vi "ziExample-Module-SweepUtility.vi"() -> ()   [LabVIEW 2016]
doc: "Control a Zurich instrument device via the LabOne Labview API. \nRequirements: Zurich Instruments MFLI, HF2 or UHFLI \nThis example shows how to start a sweeper module and retrieve data in an interactive vi.\n\n© Zurich Instruments AG, www.zhinst.com"
uses:
  <instrlib>/Zurich Instruments LabOne/Public/Modules/ziTypeModEnum.ctl
  <instrlib>/Zurich Instruments LabOne/Public/Modules/ziModSetValueBinary.vi
  <instrlib>/Zurich Instruments LabOne/Public/Modules/ziModGetDoubleData.vi
  <instrlib>/Zurich Instruments LabOne/Public/Modules/ziModGetByteArray.vi
  <instrlib>/Zurich Instruments LabOne/Public/Modules/ziModGetSweeperData.vi
  <instrlib>/Zurich Instruments LabOne/Public/Modules/ziModSetValueDouble.vi
  <instrlib>/Zurich Instruments LabOne/Zurich Instruments LabOne.lvlib
panel:
  out "Error Out":errorcluster
  in  "Host:port (optional)":string
  out "Mod subs paths":string[](array[string])
  in  "demods/x/sample":bool[](array[boolean])=[TRUE]
  in  "sweep/xmapping":i32(ring)=1 caption="X Mapping" items=["Linear", "Log"]
  in  "sweep/loopcount":i32=2 caption="Loop Count (#)" min=1 max=66000
  in  "sweep/order":u16(ring) caption="Order" items=["Current Setting", "6 dB/oct", "12 dB/oct", "18 dB/oct", "24 dB/oct", "30 dB/oct", "36 dB/oct", "42 dB/oct", "48 dB/oct"]
  out "Progress":dbl(slide) scale=0.0..1.0
  out "Finished?":bool
  in  "sweep/settling/inaccuracy":dbl caption="Inaccuracy" format="%#_5p"
  in  "sweep/scan":u16(ring) caption="Scan" items=["Sequential", "Binary", "Bidirectional"]
  in  "sweep/settling/time":dbl caption="Settling (s)" format="%#_5p"
  in  "sweep/bandwidth":dbl caption="BW (Hz)" format="%#_5p"
  in  "sweep/bandwidthcontrol":u16(ring) caption="BW Control" items=["Manual", "Fixed", "Automatic"]
  in  "sweep/phaseunwrap":bool caption="Phase Unwrap"
  in  "sweep/maxbandwidth":dbl caption="Max BW (Hz)" format="%#_5p"
  in  "sweep/averaging/tc":dbl caption="Averaging TCs" format="%#_5p"
  in  "sweep/averaging/sample":dbl caption="Averaging Samples" format="%#_5p"
  in  "Stop Sweep":bool
  in  "sweep/endless":bool caption="Endless"
  in  "start_act":bool
  in  "sweep/gridnode":string="oscs/0/freq"
  in  "sweep/omegasuppression":dbl caption="Omega Suppression (dB)" format="%#_5p"
  in  "sweep/sincfilter":bool caption="Sinc"
  in  "sweep/samplecount":i32=2 caption="Points (#)" min=2 max=66000
  in  "sweep/stop":dbl caption="Stop (Hz)" format="%_5p"
  in  "sweep/start":dbl caption="Start (Hz)" format="%_5p"
  in  "stop":bool
  in  "Address":string="DEV" caption="Device ID"
  out "Selected Device":string
  out "Sweeper Phase":cluster{"grid":dbl[], "phase":dbl[]}[](graph)
  out "Sweeper R":cluster{"grid":dbl[], "phase":dbl[]}[](graph)
  # "ziExample-SweepModul.vi\nRequirements: HF2LI, UHFLI or MFLI\nsee block diagram for VI description"
  # "Tested Devices:\n- MFLI\n- HF2LI\n- UHFLI"
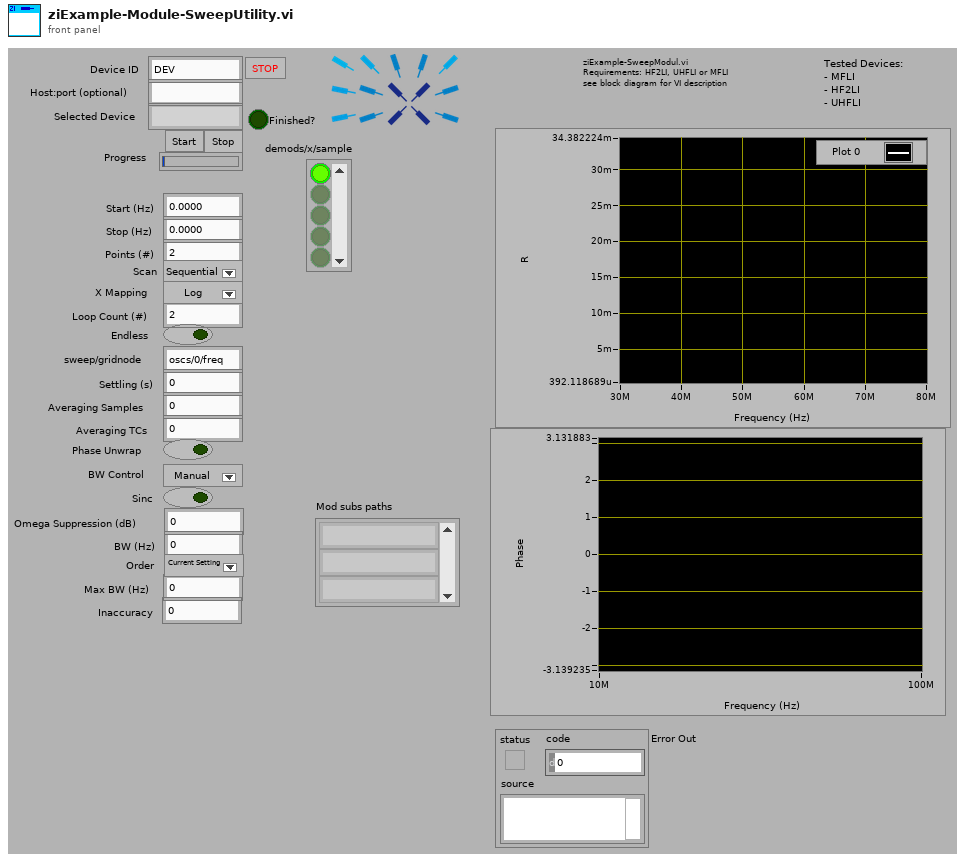
[diagram p1: front panel]
types:
  T1 = typedef "Zurich Instruments LabOne.lvlib/ziTypeModEnum.ctl" = u16
  T2 = typedef "Zurich Instruments LabOne.lvlib/ziTypeHandle.ctl" = cluster{"handleValid":bool, "Conn":u64, "Path Prefix":string, "Handle":u64, "Connected":bool, "Clockbase(s)":dbl}
  T3 = typedef "Zurich Instruments LabOne.lvlib/ziTypeModHandle.ctl" = cluster{"handleValid":bool, "Conn":u64, "ModHandle":u64, "moduleID":string, "Path Prefix":string}
  T4 = cluster{"Label.Text":string, "Label.Text 2":string}
  T5 = typedef "Zurich Instruments LabOne.lvlib/ziTypeModResults.ctl" = cluster{"PathArray":string[], "ValueType":T6, "NoOfResults":u64, "ziGenericHeader":T7[]}
  T6 = typedef "Zurich Instruments LabOne.lvlib/ziTypePollType.ctl" = enum16{"NONE", "DOUBLE_DATA", "INTEGER_DATA", "DEMOD_SAMPLE", "SCOPE_WAVE_HF2", "AUXIN_SAMPLE", "DIO_SAMPLE", "BYTE_ARRAY", "PWA_WAVE", "9", "10", "11", "12", "13", "14", "15", "TREE_CHANGE_DEPRI", "17", "ERROR", "19", "20", "21", "22", "23", "24", "25", "26", "27", "28", "29", "30", "31", "DOUBLE_DATA_TS", "INTEGER_DATA_TS", "34", "SCOPE_WAVE", "SCOPE_WAVE_EX", "37", "BYTE_ARRAY_TS", "39", "40", "41", "42", "43", "44", "45", "CNT_DATA", "47", "TREE_CHANGE", "49", "50", "51", "52", "53", "54", "55", "56", "57", "58", "59", "60", "61", "62", "63", "SWEEPER_DATA", "SPECTRUM_DATA", "ADVISOR_DATA", "VECTOR_DATA", "IMP_DATA"}
  T7 = typedef "Zurich Instruments LabOne.lvlib/ziTypeModGenericHeader.ctl" = cluster{"HeaderType":enum8{"HEADER_TYPE_NONE", "HEADER_TYPE_SWTRIGGER", "HEADER_TYPE_SWEEPER"}, "SampleFormat":u8, "SystemTime":timestamp, "CreatedTimeStamp":u64, "ChangedTimeStamp":u64, "Flags":u32, "ChunkSizeBytes":u64, "Name":string, "Status":u32, "GroupIndex":u32, "Color":u32, "ActiveRow":u32, "TriggerNumber":u64, "GridRows":u32, "GridCols":u32, "GridMode":u32, "GridOperation":u32, "GridDirection":u32, "GridRepetitions":u32, "GridColDelta":dbl, "GridColOffset":dbl, "GridRowDelta":dbl, "GridRowOffset":dbl, "Bandwidth":dbl, "Center":dbl, "Nenbw":dbl}
  T8 = typedef "Zurich Instruments LabOne.lvlib/ziTypeByteArray.ctl" = cluster{"Timestamp (ticks)":u64[], "string":string[]}
  T9 = typedef "Zurich Instruments LabOne.lvlib/ziTypeModSweeperDemodWave.ctl" = cluster{"timestamp":u64, "sampleCount":u64, "flags":u8, "sampleFormat":u8, "sweepMode":u8, "bandwidthMode":u8, "count":u64[], "settimestamp":u64[], "nexttimestamp":u64[], "grid":dbl[], "bandwidth":dbl[], "tc":dbl[], "tcmeas":dbl[], "settling":dbl[], "x":dbl[], "xstddev":dbl[], "xpwr":dbl[], "y":dbl[], "ystddev":dbl[], "ypwr":dbl[], "r":dbl[], "rstddev":dbl[], "rpwr":dbl[], "phase":dbl[], "phasestddev":dbl[], "phasepwr":dbl[], "frequency":dbl[], "frequencystddev":dbl[], "frequencypwr":dbl[], "auxin0":dbl[], "auxin0stddev":dbl[], "auxin0pwr":dbl[], "auxin1":dbl[], "auxin1stddev":dbl[], "auxin1pwr":dbl[]}
  T10 = cluster{"Label.Text":string, "Label.Text 2":string}[]
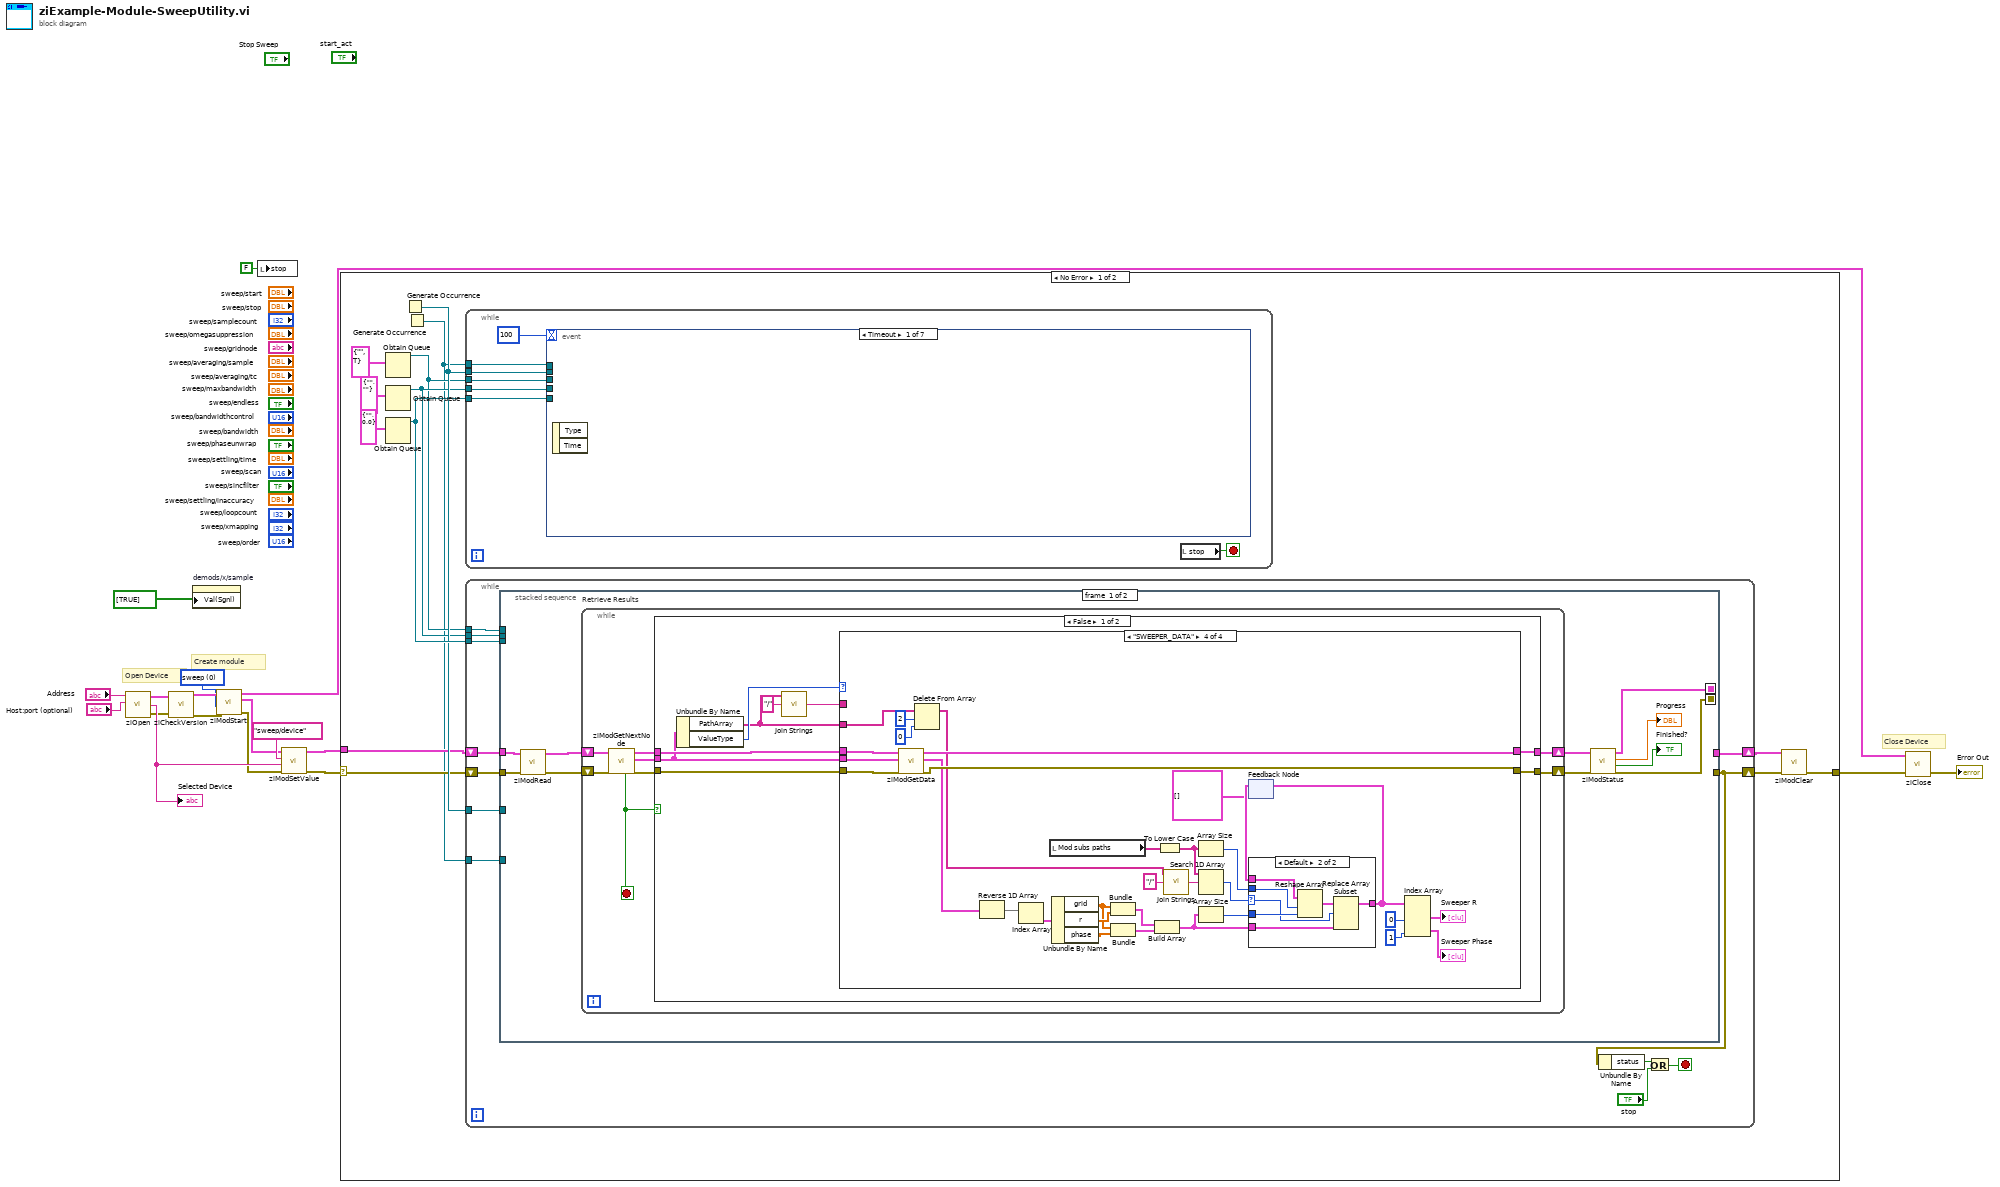
[diagram p0: block diagram]
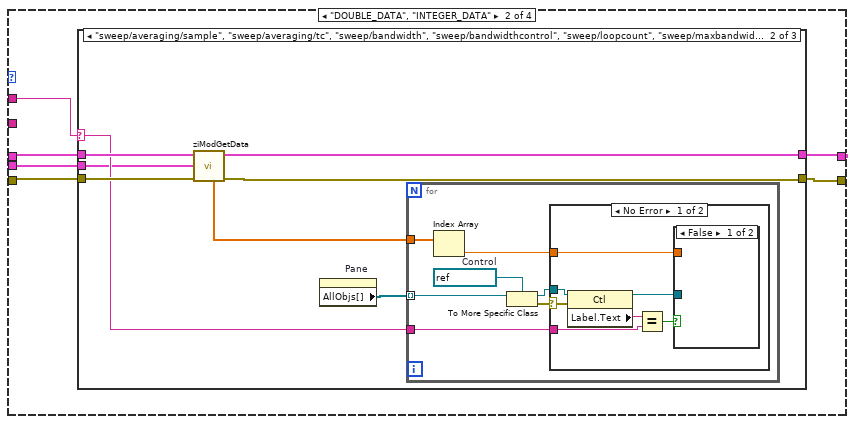
[diagram p3: hidden frame]
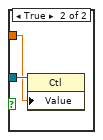
[diagram p5: hidden frame]
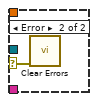
[diagram p6: hidden frame]
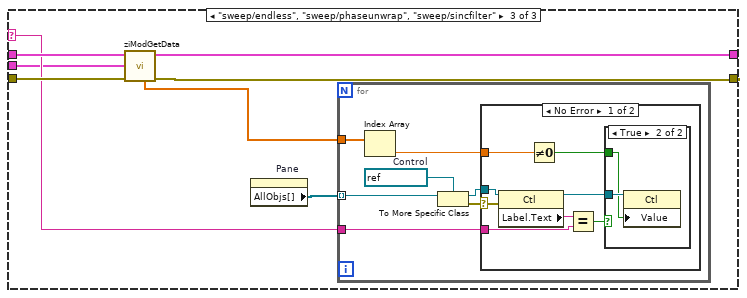
[diagram p7: hidden frame]
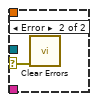
[diagram p9: hidden frame]
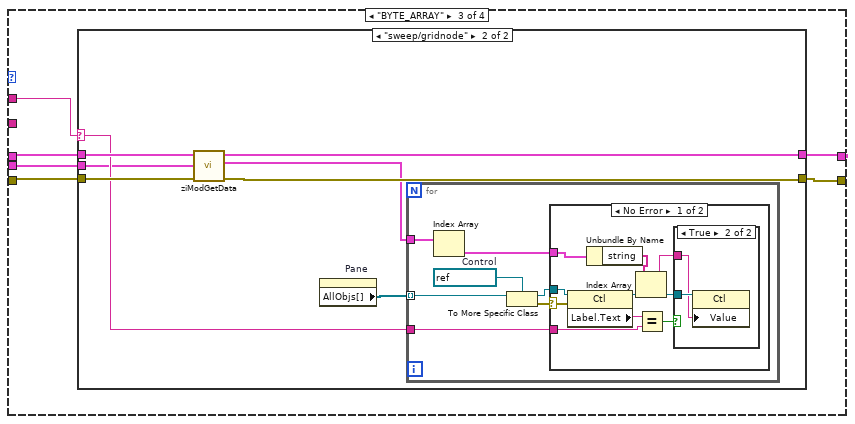
[diagram p10: hidden frame]
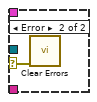
[diagram p13: hidden frame]
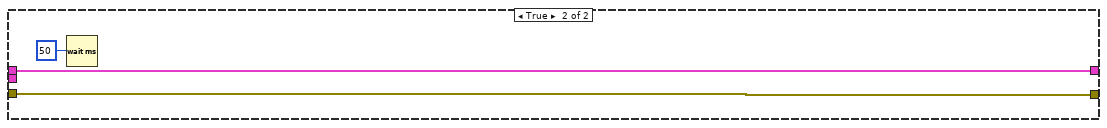
[diagram p15: hidden frame]
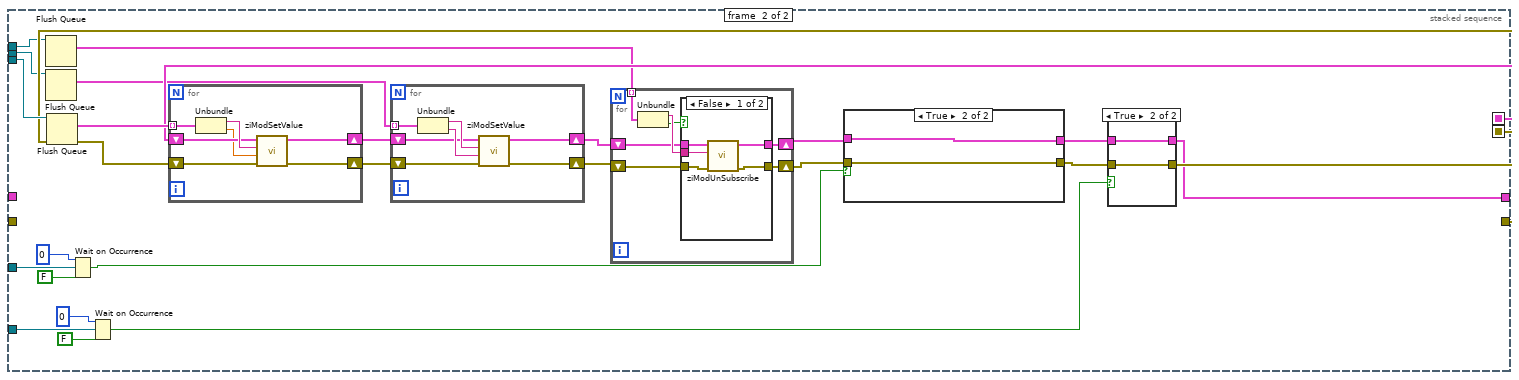
[diagram p16: hidden frame]
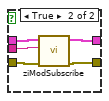
[diagram p17: hidden frame]
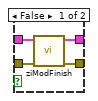
[diagram p18: hidden frame]
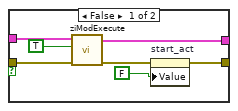
[diagram p19: hidden frame]
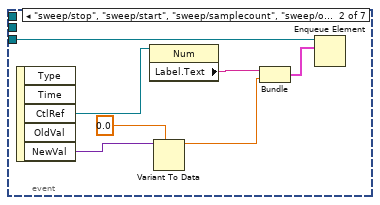
[diagram p20: hidden frame]
diagram:
  w1 = T1 0 items=["sweep", "scopeModule", "dataAcquisitionModule", "pidAdvisor", "awgModule", "impedanceModule", "multiDeviceSyncModule", "zoomFFT", "trigger", "deviceSettings", "record"] ("module Id")
  # "Close Device"
  # "Create module"
  # "Open Device"
  n1 = call <instrlib>:"ziOpen.vi"("Hostname obsolete (auto)"="Host:port (optional)", "Address"="Address") -> ("Error Out"=w5:errorcluster, "Selected Device"=w17:string, "HandleOut"=w6:T2)  [unwired: 1 in, 1 out]
  "Selected Device" <- w17
  n2 = call <instrlib>:"ziCheckVersion.vi"("Handle In"=w6, "Error In"=w5) -> ("Handle Out"=w4:T2, "Error Out"=w3:errorcluster)  [unwired: 11 in, 1 out]
  n3 = property on="demods/x/sample" class="Arr (strict)"("Val(Sgnl)"=bool[] [TRUE] ("Value (Signaling)")) -> ()  [unwired: 2 in, 2 out]
  n4 = call <instrlib>:"ziModStart.vi"("Error In"=w3, "module Id"=w1, "Handle In"=w4) -> ("Error Out"=w15:errorcluster, "ModHandle Out"=w13:T3, "Handle Out"=w16:T2)  [unwired: 6 in]
  n5 = local write "stop"(FALSE ("Stop")) -> ()
  n6 = call-poly <instrlib>:"ziModSetValue.vi"("Error In"=w15, "Data"=w17, "Path"="sweep/device", "ModHandle In"=w13) -> ("Error Out"=w10:errorcluster, "ModHandle Out"=w12:T3)  [unwired: 6 in]
  n7 = case shown="No Error" w10 {
    selector: w10 -> [w24 w329]
    tunnel: [w31 w329] -> w18
    tunnel: w12 -> [w25 _]
    frame No Error {
      n8 = Obtain Queue(element data type=cluster{"Label.Text":string, bool} {"Label.Text"="", TRUE} ("output cluster")) -> (queue out=w20:refnum<queue>)  [unwired: 4 in, 2 out]
      n9 = Obtain Queue(element data type=T4 {"Label.Text"="", "Label.Text 2"=""} ("output cluster")) -> (queue out=w21:refnum<queue>)  [unwired: 4 in, 2 out]
      n10 = Obtain Queue(element data type=cluster{"Label.Text":string, "sweep/stop":dbl} {"Label.Text"="", "sweep/stop"=0.0} ("output cluster")) -> (queue out=w27:refnum<queue>)  [unwired: 4 in, 2 out]
      n11 = Generate Occurrence() -> (w26:refnum<k4>)
      n12 = Generate Occurrence() -> (w19:refnum<k4>)
      n13 = while {
        tunnel: w27 -> [w287]
        tunnel: w26 -> [w286]
        tunnel: w21 -> [w285]
        tunnel: w20 -> [w284]
        tunnel: w19 -> [w283]
        stop <- w289 stop-if-true
        n14 = event shown="[0] Timeout" {
          selector: _ -> [_ _ _ _ _ _ _]
          dyn-events: _ -> [_ _ _ _ _ _ _]
          timeout: 100 -> [_ _ _ _ _ _ _]
          tunnel: w287 -> [_ w293 w297 _ _ _ _]
          tunnel: w286 -> [_ _ _ _ w310 _ _]
          tunnel: w285 -> [_ _ _ w307 _ _ _]
          tunnel: w284 -> [_ _ _ _ _ w311 _]
          tunnel: w283 -> [_ _ _ _ _ _ w328]
          event Timeout {
            n15 = event-data() -> ()  [unwired: 1 in, 2 out]
          }
          event "sweep/stop", "sweep/start", "sweep/samplecount", "sweep/omegasuppression", "sweep/averaging/sample", "sweep/averaging/tc", "sweep/maxbandwidth", "sweep/bandwidthcontrol", "sweep/settling/time", "sweep/scan", "sweep/loopcount", "sweep/xmapping", "sweep/order": Value Change {
            n16 = event-data() -> ("CtlRef"=w294:refnum<vi>, "NewVal"=w295:variant)  [unwired: 1 in, 3 out]
            n17 = property class="Num"(reference=w294) -> ("Label.Text"=w292:string)  [unwired: 1 in, 2 out]
            n18 = Variant To Data(type=0.0 ("sweep/stop"), Variant=w295) -> (data=w291:dbl)  [unwired: 1 in, 1 out]
            n19 = Bundle("Label.Text"=w292, "sweep/stop"=w291) -> (w290:cluster{"Label.Text":string, "sweep/stop":dbl})  [unwired: 1 in]
            n20 = Enqueue Element(queue=w293, element=w290) -> ()  [unwired: 2 in, 3 out]
          }
          event "sweep/phaseunwrap", "sweep/endless", "sweep/sincfilter": Value Change {
            n21 = event-data() -> ("CtlRef"=w302:refnum<vi>, "NewVal"=w299:bool)  [unwired: 1 in, 3 out]
            n22 = property class="Bool (strict)"(reference=w302) -> ("Label.Text"=w301:string)  [unwired: 1 in, 2 out]
            n23 = Boolean To (0,1)(Boolean=w299) -> (0, 1=w300:i16)
            n24 = Bundle("Label.Text"=w301, w300) -> (w298:cluster{"Label.Text":string, i16})  [unwired: 1 in]
            n25 = Enqueue Element(queue=w297, element=w298) -> ()  [unwired: 2 in, 3 out]
          }
          event "sweep/gridnode": Value Change {
            n26 = event-data() -> ("CtlRef"=w309:refnum<vi>, "NewVal"=w303:string)  [unwired: 1 in, 3 out]
            n27 = property class="Str"(reference=w309) -> ("Label.Text"=w304:string)  [unwired: 1 in, 2 out]
            n28 = Variant To Data(type="", Variant=w303) -> (data=w308:string)  [unwired: 1 in, 1 out]
            n29 = Bundle("Label.Text"=w304, w308) -> (w305:cluster{"Label.Text":string, string})  [unwired: 1 in]
            n30 = Enqueue Element(queue=w307, element=w305) -> ()  [unwired: 2 in, 3 out]
          }
          event "start_act": Value Change {
            n31 = event-data() -> ()  [unwired: 1 in, 5 out]
            n32 = Set Occurrence(w310) -> ()
          }
          event "demods/x/sample": Value Change {
            n33 = event-data() -> ()  [unwired: 1 in, 5 out]
            n34 = for {
              tunnel: "demods/x/sample" -> [w320] mode=indexing
              tunnel: "demods/%d/sample" -> [w319]
              shift-right: [w321] -> w312
              shift-left: string[] [] ("Mod subs paths") -> [w322]
              tunnel: w311 -> [w317]
              i -> [w323]
              n35 = Format Into String(format string=w319, w323) -> (resulting string=w316:string)  [unwired: 2 in, 1 out]
              n36 = Bundle(w316, "Boolean"=w320) -> (w318:cluster{string, "Boolean":bool})  [unwired: 1 in]
              n37 = case shown="False" w320 {
                tunnel: w322 -> [w324 w327]
                tunnel: w316 -> [_ w326]
                tunnel: [w324 w325] -> w321
                frame False {
                }
                frame True {
                  n38 = Build Array (concatenate)(w327, w326) -> (w325:string[])
                }
              }
              n39 = Enqueue Element(queue=w317, element=w318) -> ()  [unwired: 2 in, 3 out]
            }
            "Mod subs paths" <- w312
          }
          event "Stop Sweep": Value Change {
            n40 = event-data() -> ()  [unwired: 1 in, 5 out]
            n41 = Set Occurrence(w328) -> ()
          }
        }
        n42 = local read "stop"() -> (w289:bool)
      }
      n43 = while {
        shift-right: [w36] -> w30
        shift-left: w25 -> [w40]
        shift-right: [w35] -> w29
        shift-left: w24 -> [w43]
        tunnel: w27 -> [w42]
        tunnel: w26 -> [w41]
        tunnel: w21 -> [w39]
        tunnel: w20 -> [w38]
        tunnel: w19 -> [w37]
        stop <- w32 stop-if-true
        n44 = stacked-sequence {
          seq-local: [w46 _] -> [_ w230]
          seq-local: [w44 _] -> [_ w229]
          tunnel: w43 -> [w53 _]
          tunnel: w42 -> [_ w236]
          tunnel: w41 -> [_ w234]
          tunnel: w40 -> [w45 _]
          tunnel: w39 -> [_ w227]
          tunnel: w38 -> [_ w226]
          tunnel: w37 -> [_ w216]
          tunnel: [_ w212] -> w35
          tunnel: [_ w211] -> w36
          frame #0 {
            n45 = call <instrlib>:"ziModRead.vi"("error in"=w53, "ziModHandle In"=w45) -> ("error out"=w52:errorcluster, "ziModHandle Out"=w51:T3)  [unwired: 8 in]
            n46 = while "Retrieve Results" {
              shift-right: [w58] -> w50
              shift-left: w51 -> [w60]
              shift-right: [w57] -> w48
              shift-left: w52 -> [w61]
              stop <- w54 stop-if-true
              n47 = call <instrlib>:"ziModGetNextNode.vi"("Error In"=w61, "ModHandle In"=w60) -> ("Error Out"=w55:errorcluster, "ModResults"=w56:T5, "ModHandle Out"=w59:T3, "NoData"=w54:bool)  [unwired: 6 in]
              n48 = case shown="False" w54 {
                tunnel: w59 -> [w70 w207]
                tunnel: [w69 w207] -> w58
                tunnel: [w68 w208] -> w57
                tunnel: w56 -> [w66 _]
                tunnel: w55 -> [w65 w208]
                frame False {
                  n49 = Unbundle By Name(w66) -> ("PathArray"=w64:string[], "ValueType"=w67:T6)
                  n50 = call <vilib>:"Join Strings.vi"("Separator (,)"="/", "Strings In"=w64) -> ("String"=w62:string)  [unwired: 1 in]
                  n51 = case shown="\"SWEEPER_DATA\"" w67 {
                    tunnel: w70 -> [w72 w78 w137 w198]
                    tunnel: w66 -> [_ w73 w132 w179]
                    tunnel: w65 -> [w71 w77 w136 w197]
                    tunnel: [w72 w76 w135 w195] -> w69
                    tunnel: [w71 w75 w134 w196] -> w68
                    tunnel: w64 -> [_ _ _ w171]
                    tunnel: w62 -> [_ w74 w133 _]
                    frame "NONE", Default {
                    }
                    frame "DOUBLE_DATA", "INTEGER_DATA" {
                      n52 = case shown="\"sweep/averaging/sample\", \"sweep/averaging/tc\", \"sweep/bandwidth\", \"sweep/bandwidthcontrol\", \"sweep/loopcount\", \"sweep/maxbandwidth\", \"sweep/omegasuppression\", \"sweep/order\", \"sweep/remainingtime\", \"sweep/samplecount\", \"sweep/scan\", \"sweep/settling/inaccuracy\", \"sweep/settling/time\", \"sweep/start\", \"sweep/stop\", \"sweep/xmapping\"" w74 {
                        selector: w74 -> [_ w82 w107]
                        tunnel: w78 -> [w80 w88 w113]
                        tunnel: w77 -> [w79 w85 w110]
                        tunnel: [w79 w86 w111] -> w75
                        tunnel: [w80 w87 w112] -> w76
                        tunnel: w73 -> [_ w81 w106]
                        frame Default {
                        }
                        frame "sweep/averaging/sample", "sweep/averaging/tc", "sweep/bandwidth", "sweep/bandwidthcontrol", "sweep/loopcount", "sweep/maxbandwidth", "sweep/omegasuppression", "sweep/order", "sweep/remainingtime", "sweep/samplecount", "sweep/scan", "sweep/settling/inaccuracy", "sweep/settling/time", "sweep/start", "sweep/stop", "sweep/xmapping" {
                          n53 = call-poly <instrlib>:"ziModGetData.vi"("Error In"=w85, "ModResults"=w81, "ModHandle In"=w88) -> ("Error Out"=w86:errorcluster, "ModHandle Out"=w87:T3, "Value"=w83:dbl[])  [unwired: 4 in, 2 out]
                          n54 = property on="Pane" class="Pane"() -> ("AllObjs[]"=w84:refnum<vi>[])  [unwired: 2 in, 2 out]
                          n55 = for {
                            tunnel: w84 -> [w93] mode=indexing
                            tunnel: w82 -> [w92]
                            tunnel: w83 -> [w89]
                            w95 = refnum<vi> refnum  # Control
                            n56 = Index Array(array=w89) -> (element=w90:dbl)  [unwired: 1 in]
                            n57 = To More Specific Class(target class=w95, reference=w93) -> (specific class reference=w94:refnum<vi>, error out=w91:errorcluster)  [unwired: 1 in]
                            n58 = case shown="No Error" w91 {
                              selector: w91 -> [w96 w105]
                              tunnel: w94 -> [w102 _]
                              tunnel: w92 -> [w100 _]
                              tunnel: w90 -> [w97 _]
                              frame No Error {
                                n59 = property class="Ctl"(reference=w102, error in=w96) -> (reference out=w98:refnum<vi>, "Label.Text"=w101:string)  [unwired: 1 out]
                                n60 = Equal?(x=w101, y=w100) -> (x = y?=w99:bool)
                                n61 = case shown="False" w99 {
                                tunnel: w98 -> [_ w104]
                                tunnel: w97 -> [_ w103]
                                frame False {
                                }
                                frame True {
                                n62 = property class="Ctl"(reference=w104, "Value"=w103) -> ()  [unwired: 1 in, 2 out]
                                }
                                }
                              }
                              frame Error {
                                n63 = call <vilib>:"Clear Errors.vi"("error in (no error)"=w105) -> ()  [unwired: 5 in, 2 out]
                              }
                            }
                          }
                        }
                        frame "sweep/endless", "sweep/phaseunwrap", "sweep/sincfilter" {
                          n64 = call-poly <instrlib>:"ziModGetData.vi"("Error In"=w110, "ModResults"=w106, "ModHandle In"=w113) -> ("Error Out"=w111:errorcluster, "ModHandle Out"=w112:T3, "Value"=w108:dbl[])  [unwired: 4 in, 2 out]
                          n65 = property on="Pane" class="Pane"() -> ("AllObjs[]"=w109:refnum<vi>[])  [unwired: 2 in, 2 out]
                          n66 = for {
                            tunnel: w109 -> [w118] mode=indexing
                            tunnel: w107 -> [w117]
                            tunnel: w108 -> [w114]
                            w120 = refnum<vi> refnum  # Control
                            n67 = Index Array(array=w114) -> (element=w115:dbl)  [unwired: 1 in]
                            n68 = To More Specific Class(target class=w120, reference=w118) -> (specific class reference=w119:refnum<vi>, error out=w116:errorcluster)  [unwired: 1 in]
                            n69 = case shown="No Error" w116 {
                              selector: w116 -> [w123 w131]
                              tunnel: w119 -> [w128 _]
                              tunnel: w117 -> [w126 _]
                              tunnel: w115 -> [w122 _]
                              frame No Error {
                                n70 = property class="Ctl"(reference=w128, error in=w123) -> (reference out=w124:refnum<vi>, "Label.Text"=w127:string)  [unwired: 1 out]
                                n71 = Not Equal To 0?(x=w122) -> (x != 0?=w121:bool)
                                n72 = Equal?(x=w127, y=w126) -> (x = y?=w125:bool)
                                n73 = case shown="True" w125 {
                                tunnel: w124 -> [_ w130]
                                tunnel: w121 -> [_ w129]
                                frame False {
                                }
                                frame True {
                                n74 = property class="Ctl"(reference=w130, "Value"=w129) -> ()  [unwired: 1 in, 2 out]
                                }
                                }
                              }
                              frame Error {
                                n75 = call <vilib>:"Clear Errors.vi"("error in (no error)"=w131) -> ()  [unwired: 5 in, 2 out]
                              }
                            }
                          }
                        }
                      }
                    }
                    frame "BYTE_ARRAY" {
                      n76 = case shown="\"sweep/gridnode\"" w133 {
                        selector: w133 -> [_ w142]
                        tunnel: w137 -> [w139 w147]
                        tunnel: w136 -> [w138 w144]
                        tunnel: [w138 w145] -> w134
                        tunnel: [w139 w146] -> w135
                        tunnel: w132 -> [_ w141]
                        frame Default {
                        }
                        frame "sweep/gridnode" {
                          n77 = call-poly <instrlib>:"ziModGetData.vi"("Error In"=w144, "ModResults"=w141, "ModHandle In"=w147) -> ("Error Out"=w145:errorcluster, "ByteArray"=w140:T8[], "ModHandle Out"=w146:T3)  [unwired: 6 in]
                          n78 = property on="Pane" class="Pane"() -> ("AllObjs[]"=w143:refnum<vi>[])  [unwired: 2 in, 2 out]
                          n79 = for {
                            tunnel: w143 -> [w152] mode=indexing
                            tunnel: w142 -> [w151]
                            tunnel: w140 -> [w149]
                            w154 = refnum<vi> refnum  # Control
                            n80 = Index Array(array=w149) -> (element=w148:T8)  [unwired: 1 in]
                            n81 = To More Specific Class(target class=w154, reference=w152) -> (specific class reference=w153:refnum<vi>, error out=w150:errorcluster)  [unwired: 1 in]
                            n82 = case shown="No Error" w150 {
                              selector: w150 -> [w158 w166]
                              tunnel: w153 -> [w163 _]
                              tunnel: w151 -> [w161 _]
                              tunnel: w148 -> [w157 _]
                              frame No Error {
                                n83 = property class="Ctl"(reference=w163, error in=w158) -> (reference out=w159:refnum<vi>, "Label.Text"=w162:string)  [unwired: 1 out]
                                n84 = Unbundle By Name(w157) -> ("string"=w156:string[])
                                n85 = Index Array(array=w156) -> (element=w155:string)  [unwired: 1 in]
                                n86 = Equal?(x=w162, y=w161) -> (x = y?=w160:bool)
                                n87 = case shown="True" w160 {
                                tunnel: w159 -> [_ w165]
                                tunnel: w155 -> [_ w164]
                                frame False {
                                }
                                frame True {
                                n88 = property class="Ctl"(reference=w165, "Value"=w164) -> ()  [unwired: 1 in, 2 out]
                                }
                                }
                              }
                              frame Error {
                                n89 = call <vilib>:"Clear Errors.vi"("error in (no error)"=w166) -> ()  [unwired: 5 in, 2 out]
                              }
                            }
                          }
                        }
                      }
                    }
                    frame "SWEEPER_DATA" {
                      n90 = call-poly <instrlib>:"ziModGetData.vi"("Error In"=w197, "ModResults"=w179, "ModHandle In"=w198) -> ("Error Out"=w196:errorcluster, "SweeperDemodWaveArray"=w182:T9[], "ModHandle Out"=w195:T3)  [unwired: 4 in, 2 out]
                      n91 = Delete From Array(array=w171, length=2 ("index"), index=0) -> (array with subset deleted=w168:string[])  [unwired: 1 out]
                      n92 = Reverse 1D Array(array=w182) -> (reversed array=w181:T9[])
                      n93 = Index Array(array=w181) -> (element=w191:T9)  [unwired: 1 in]
                      n94 = local read "Mod subs paths"() -> (w173:string[])
                      n95 = Unbundle By Name(w191) -> ("grid"=w192:dbl[], "r"=w194:dbl[], "phase"=w193:dbl[])
                      n96 = Bundle("grid"=w192, "r"=w194) -> (w187:cluster{"grid":dbl[], "r":dbl[]})  [unwired: 1 in]
                      n97 = Bundle("grid"=w192, "phase"=w193) -> (w180:cluster{"grid":dbl[], "phase":dbl[]})  [unwired: 1 in]
                      n98 = Build Array(w187, w180) -> (w178:cluster{"grid":dbl[], "phase":dbl[]}[])
                      n99 = To Lower Case(string=w173) -> (all lower case string=w172:string[])
                      n100 = call <vilib>:"Join Strings.vi"("Separator (,)"="/", "Strings In"=w168) -> ("String"=w169:string)  [unwired: 1 in]
                      n101 = Array Size(array=w172) -> (size(s)=w188:i32)
                      n102 = Search 1D Array(1D array=w172, element=w169) -> (index of element=w175:i32)  [unwired: 1 in]
                      n103 = Array Size(array=w178) -> (size(s)=w177:i32)
                      n104 = feedback #1(cluster{"grid":dbl[], "phase":dbl[]}[][] []) -> (w186:cluster{"grid":dbl[], "phase":dbl[]}[][])
                      n105 = case shown="Default" w175 {
                        selector: w175 -> [_ w200]
                        tunnel: w188 -> [_ w206]
                        tunnel: w186 -> [w199 w204]
                        tunnel: [w199 w203] -> w185
                        tunnel: w178 -> [_ w202]
                        tunnel: w177 -> [_ w201]
                        frame -1 {
                        }
                        frame Default {
                          n106 = Reshape Array(w204, w206, w201) -> (w205:cluster{"grid":dbl[], "phase":dbl[]}[][])
                          n107 = Replace Array Subset(array=w205, new element=w202, index (row)=w200) -> (w203:cluster{"grid":dbl[], "phase":dbl[]}[][])  [unwired: 1 in]
                        }
                      }
                      n108 = feedback-in #1(w185) -> ()
                      n109 = Index Array(array=w185, index (col) #1=0 ("disabled index (col)"), index (col) #2=1 ("index (col)")) -> (element #1=→"Sweeper R":cluster{"grid":dbl[], "phase":dbl[]}[], element #2=→"Sweeper Phase":cluster{"grid":dbl[], "phase":dbl[]}[])  [unwired: 2 in]
                    }
                  }
                }
                frame True {
                  n110 = Wait (ms)(milliseconds to wait=u32 50) -> ()  [unwired: 1 out]
                }
              }
            }
            n111 = call <instrlib>:"ziModStatus.vi"("Error In"=w48, "ModHandle IN"=w50) -> ("Error Out"=w44:errorcluster, "Finished?"=→"Finished?":bool, "Progress (unity)"=→"Progress":dbl, "ModHandle Out"=w46:T3)  [unwired: 5 in]
          }
          frame #1 {
            n112 = Flush Queue(queue=w226) -> (remaining elements=w210:cluster{"Label.Text":string, bool}[])  [unwired: 1 in, 2 out]
            n113 = Flush Queue(queue=w227) -> (remaining elements=w225:T10)  [unwired: 1 in, 2 out]
            n114 = Flush Queue(queue=w236, error in (no error)=w229) -> (remaining elements=w235:cluster{"Label.Text":string, "sweep/stop":dbl}[], error out=w228:errorcluster)  [unwired: 1 out]
            n115 = Wait on Occurrence(1:FALSE ("ignore previous (T)"), 2:w234, 3:0 ("ms timeout (-1)")) -> (0:w232:bool)
            n116 = Wait on Occurrence(1:FALSE ("ignore previous (T)"), 2:w216, 3:0 ("ms timeout (-1)")) -> (0:w215:bool)
            n117 = for {
              tunnel: w235 -> [w280] mode=indexing
              shift-right: [w279] -> w224
              shift-left: w230 -> [w281]
              shift-right: [w276] -> w223
              shift-left: w228 -> [w277]
              n118 = Unbundle(w280) -> ("Label.Text"=w282:string, "sweep/stop"=w278:dbl)
              n119 = call-poly <instrlib>:"ziModSetValue.vi"("Error In"=w277, "Value"=w278, "Path"=w282, "ModHandle In"=w281) -> ("Error Out"=w276:errorcluster, "ModHandle Out"=w279:T3)  [unwired: 6 in]
            }
            n120 = for {
              tunnel: w225 -> [w266] mode=indexing
              shift-right: [w264] -> w222
              shift-left: w224 -> [w262]
              shift-right: [w260] -> w221
              shift-left: w223 -> [w261]
              n121 = Unbundle(w266) -> ("Label.Text"=w263:string, "Label.Text 2"=w265:string)
              n122 = call-poly <instrlib>:"ziModSetValue.vi"("Error In"=w261, "Data"=w265, "Path"=w263, "ModHandle In"=w262) -> ("Error Out"=w260:errorcluster, "ModHandle Out"=w264:T3)  [unwired: 6 in]
            }
            n123 = for {
              shift-right: [w239] -> w219
              shift-left: w221 -> [w240]
              shift-right: [w238] -> w220
              shift-left: w222 -> [w241]
              tunnel: w210 -> [w237] mode=indexing
              n124 = Unbundle(w237) -> ("Label.Text"=w243:string, w242:bool)
              n125 = case shown="False" w242 {
                tunnel: w243 -> [w248 w253]
                tunnel: w241 -> [w245 w252]
                tunnel: w240 -> [w247 w251]
                tunnel: [w246 w250] -> w239
                tunnel: [w244 w249] -> w238
                frame False {
                  n126 = call <instrlib>:"ziModUnSubscribe.vi"("Error In"=w247, "Path (\"/\")"=w248, "ModHandle In"=w245) -> ("Error Out"=w246:errorcluster, "ModHandle Out"=w244:T3)  [unwired: 7 in]
                }
                frame True {
                  n127 = call <instrlib>:"ziModSubscribe.vi"("Error In"=w251, "Path"=w253, "ModHandle In"=w252) -> ("Error Out"=w250:errorcluster, "ModHandle Out"=w249:T3)  [unwired: 6 in]
                }
              }
            }
            n128 = case shown="True" w232 {
              tunnel: w220 -> [w272 w275]
              tunnel: [w271 w275] -> w214
              tunnel: w219 -> [w269 w274]
              tunnel: [w267 w274] -> w213
              frame False {
                n129 = call <instrlib>:"ziModExecute.vi"("Error In"=w269, "Modal (F)"=TRUE ("Modal"), "ziModHandle In"=w272) -> ("Error Out"=w268:errorcluster, "ziModHandle Out"=w271:T3)  [unwired: 5 in, 1 out]
                n130 = property on="start_act" class="Bool (strict)"(error in=w268, "Value"=FALSE) -> (error out=w267:errorcluster)  [unwired: 1 in, 1 out]
              }
              frame True {
              }
            }
            n131 = case shown="True" w215 {
              tunnel: w214 -> [w257 w259]
              tunnel: [w255 w259] -> w211
              tunnel: w213 -> [w256 w258]
              tunnel: [w254 w258] -> w212
              frame False {
                n132 = call <instrlib>:"ziModFinish.vi"("Error In"=w256, "ziModHandle In"=w257) -> ("Error Out"=w254:errorcluster, "ziModHandle Out"=w255:T3)  [unwired: 7 in]
              }
              frame True {
              }
            }
          }
        }
        n133 = Unbundle By Name(w35) -> ("status"=w34:bool)
        n134 = Or(x=w34, y="stop") -> (x .or. y?=w32:bool)
      }
      n135 = call <instrlib>:"ziModClear.vi"("Error In"=w29, "ziModHandle In"=w30) -> ("Error Out"=w31:errorcluster)  [unwired: 7 in, 1 out]
    }
    frame Error {
    }
  }
  n136 = call <instrlib>:"ziClose.vi"("Error In"=w18, "Handle In"=w16) -> ("Error Out"=→"Error Out":errorcluster)  [unwired: 2 in, 1 out]
